vi "Set Value.vi"(7 "TOML string":string, 8 "error in (no error)":errorcluster, 9 "start position":i32, 10 "Value":T3, 11 "Context in":T2[](array[typedef])) -> (0 "error out":errorcluster, 1 "offset past match":i32, 2 "State":T1, 3 "Context out":T2[](array[typedef]))   [LabVIEW 2019, in "BlueTOMLSerializer.lvlib"]
uses:
  BlueTOMLSerializer.lvlib
  Value.ctl
  Key-Value Pair.ctl
  Table Context.ctl
  Table Array Context.ctl
  Array Context.ctl
  State.ctl
  <vilib>/regexp/Match Regular Expression.xnode
  Value Type.ctl
  Context.ctl
panel:
  in  "Define":bool=TRUE
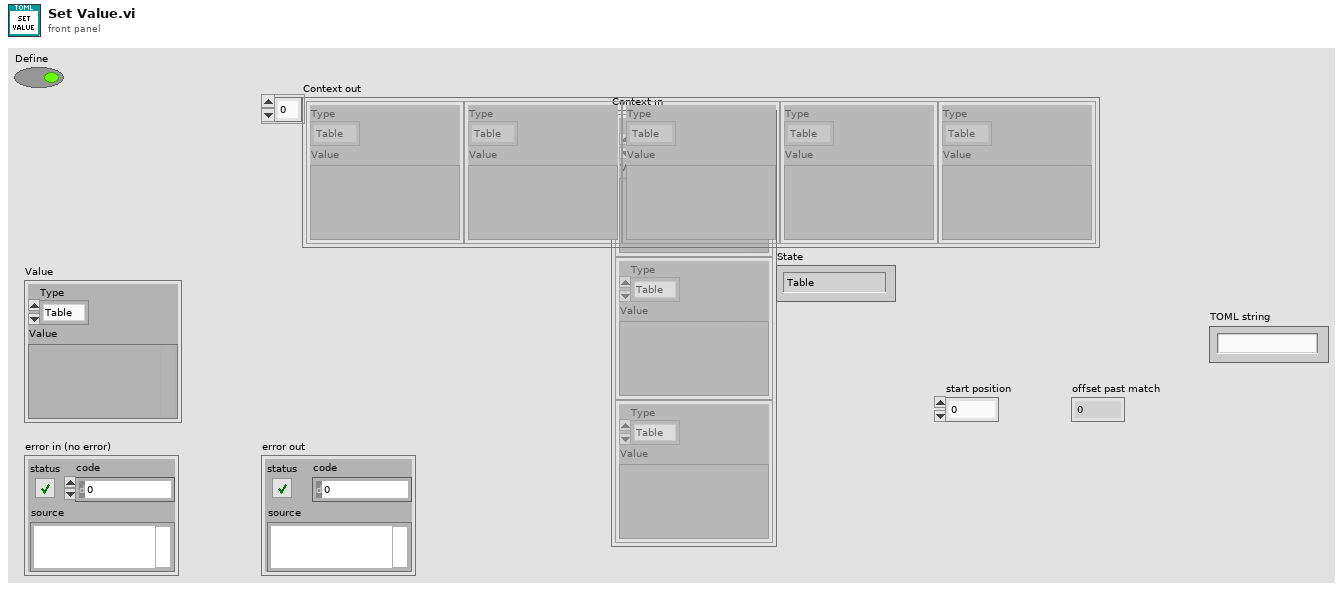
[diagram p1: front panel]
types:
  T1 = typedef "BlueTOMLSerializer.lvlib/State.ctl" = enum16{"Table", "Value", "Inline Table"}
  T2 = typedef "BlueTOMLSerializer.lvlib/Context.ctl" = cluster{"Type":enum16{"Table", "Array", "Inline Table", "Table Array"}, "Value":variant}
  T3 = typedef "BlueTOMLSerializer.lvlib/Value.ctl" = cluster{"Type":T4, "Value":variant}
  T4 = typedef "BlueTOMLSerializer.lvlib/Value Type.ctl" = enum16{"Table", "Array", "String", "Integer", "Float", "Boolean", "Offset Date-Time", "Local Date-Time", "Local Date", "Local Time"}
  T5 = typedef "BlueTOMLSerializer.lvlib/Table Context.ctl" = cluster{"Table":T6[], "Key":string, "Defined Keys":string[]}
  T6 = typedef "BlueTOMLSerializer.lvlib/Key-Value Pair.ctl" = cluster{"Key":string, "Value":T3}
  T7 = typedef "BlueTOMLSerializer.lvlib/Table Array Context.ctl" = cluster{"Table Array":cluster{"Table":T6[]}[], "Index":i32, "Key":string}
  T8 = typedef "BlueTOMLSerializer.lvlib/Array Context.ctl" = cluster{"Array":T3[], "Index":i32, "Empty":bool, "Type":T4}
  T9 = enum16{"Table", "Array", "Inline Table", "Table Array"}
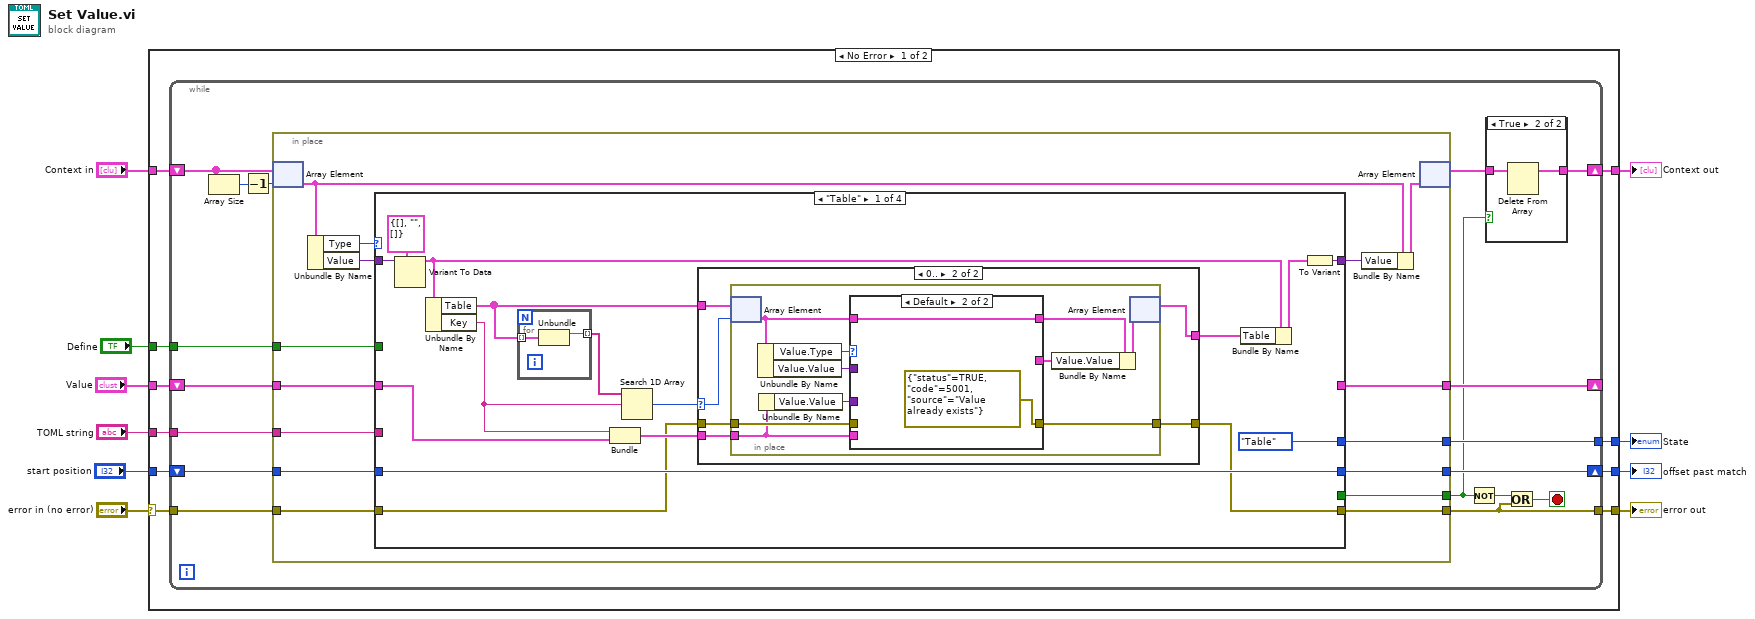
[diagram p0: block diagram]
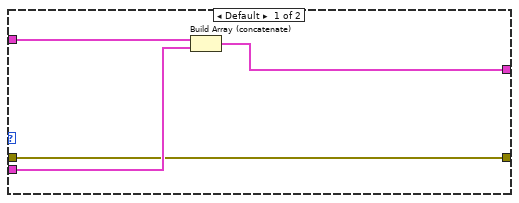
[diagram p3: hidden frame]
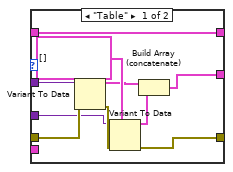
[diagram p4: hidden frame]
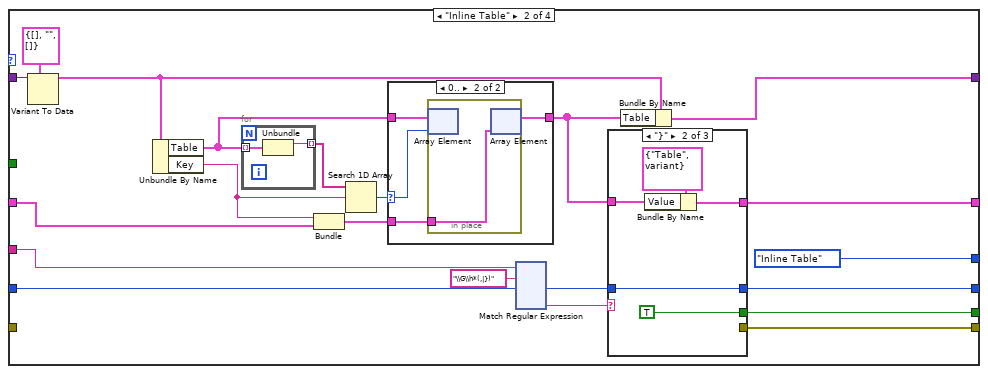
[diagram p5: hidden frame]
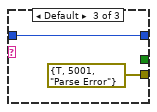
[diagram p7: hidden frame]
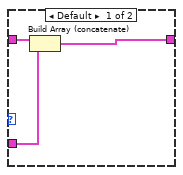
[diagram p8: hidden frame]
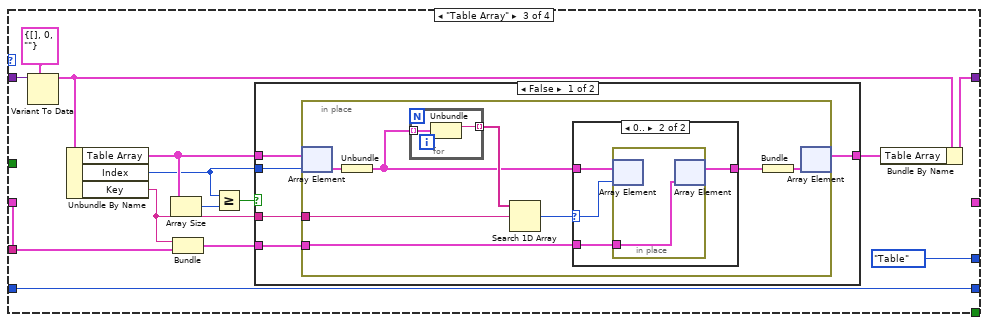
[diagram p9: hidden frame]
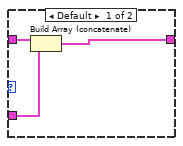
[diagram p10: hidden frame]
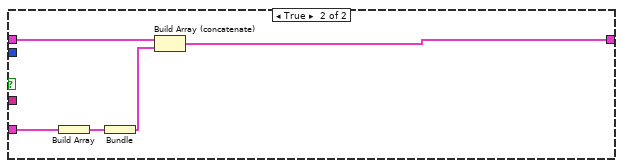
[diagram p11: hidden frame]
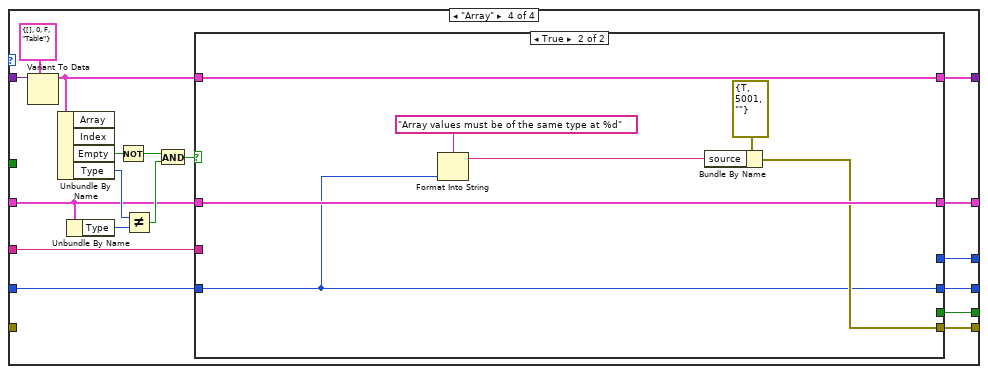
[diagram p12: hidden frame]
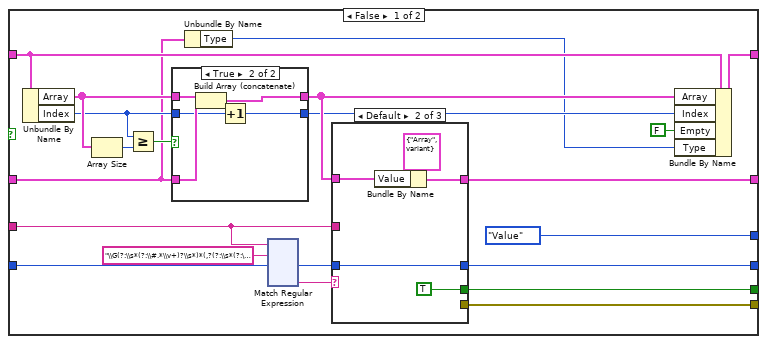
[diagram p13: hidden frame]
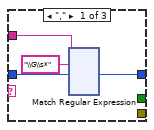
[diagram p14: hidden frame]
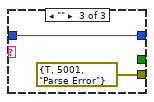
[diagram p15: hidden frame]
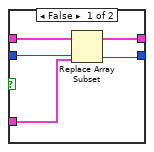
[diagram p16: hidden frame]
diagram:
  n1 = case shown="No Error" "error in (no error)" {
    selector: "error in (no error)" -> [w15 w603]
    tunnel: "Context in" -> [w20 w601]
    tunnel: [w19 w601] -> w9
    tunnel: "Value" -> [w18 _]
    tunnel: [w17 _] -> w7
    tunnel: [w16 w603] -> w6
    tunnel: "start position" -> [w14 w602]
    tunnel: "TOML string" -> [w13 _]
    tunnel: [w12 w602] -> w2
    tunnel: "Define" -> [w11 _]
    frame No Error {
      n2 = while {
        tunnel: [w33] -> w17
        tunnel: w13 -> [w28]
        shift-right: [w26] -> w12
        shift-left: w14 -> [w29]
        tunnel: w15 -> [w32]
        tunnel: [w30] -> w16
        shift-right: [w25] -> _
        shift-left: w18 -> [w34]
        shift-right: [w23] -> w19
        shift-left: w20 -> [w35]
        tunnel: w11 -> [w21]
        stop <- w31 stop-if-true
        n3 = Array Size(array=w35) -> (size(s)=w37:i32)
        n4 = Decrement(x=w37) -> (x-1=w36:i32)
        n5 = in-place {
          in-place-border: w34 -> [w50]
          in-place-border: [w49] -> w33
          in-place-border: [w48] -> w30
          in-place-border: w32 -> [w47]
          in-place-border: [w44] -> w22
          in-place-border: w29 -> [w46]
          in-place-border: w28 -> [w45]
          in-place-border: [w43] -> w25
          in-place-border: [w42] -> w26
          in-place-border: w21 -> [w41]
          n6 = in-place-array #1(w35, w36) -> (w53:T2)
          n7 = Unbundle By Name(w53) -> ("Type"=w55:T9, "Value"=w54:variant)
          n8 = case shown="\"Table\"" w55 {
            tunnel: w54 -> [w71 w126 w274 w320]
            tunnel: w50 -> [w65 w120 w270 w304]
            tunnel: [w60 w106 w263 w319] -> w52
            tunnel: [State."Table" ("State") State."Inline Table" ("State") State."Table" ("State") w317] -> w49
            tunnel: [w56 w107 _ w312] -> w48
            tunnel: w47 -> [w57 _ _ _]
            tunnel: w46 -> [w58 w116 w261 w315]
            tunnel: w45 -> [_ w115 _ w311]
            tunnel: [_ w111 _ w316] -> w44
            tunnel: [_ w109 _ w313] -> w43
            tunnel: [w58 w108 w261 w314] -> w42
            tunnel: w41 -> [_ _ _ _]
            frame "Table" {
              n9 = Variant To Data(type=T5 {"Table"=[], "Key"="", "Defined Keys"=[]} ("Table Context"), Variant=w71) -> (data=w64:T5)  [unwired: 1 in, 1 out]
              n10 = Unbundle By Name(w64) -> ("Table"=w67:T6[], "Key"=w66:string)
              n11 = for {
                tunnel: w67 -> [w105] mode=indexing
                tunnel: [w104] -> w69 mode=indexing
                n12 = Unbundle(w105) -> ("Key"=w104:string)  [unwired: 1 out]
              }
              n13 = Bundle("Key"=w66, "Value"=w65) -> (w61:cluster{"Key":string, "Value":T3})  [unwired: 1 in]
              n14 = Search 1D Array(1D array=w69, element=w66) -> (index of element=w68:i32)  [unwired: 1 in]
              n15 = case shown="0.." w68 {
                selector: w68 -> [_ w79]
                tunnel: w67 -> [w75 w81]
                tunnel: [w74 w80] -> w63
                tunnel: w61 -> [w73 w78]
                tunnel: w57 -> [w72 w77]
                tunnel: [w72 w76] -> w56
                frame Default {
                  n16 = Build Array (concatenate)(w75, w73) -> (w74:T6[])
                }
                frame 0.. {
                  n17 = in-place {
                    in-place-border: w78 -> [w84]
                    in-place-border: w77 -> [w86]
                    in-place-border: [w85] -> w76
                    n18 = in-place-array #2(w81, w79) -> (w90:T6)
                    n19 = Unbundle By Name(w90) -> ("Value.Type"=w89:T4, "Value.Value"=w88:variant)
                    n20 = Unbundle By Name(w84) -> ("Value.Value"=w83:variant)
                    n21 = case shown="Default" w89 {
                      tunnel: [w101 w103] -> w91
                      tunnel: w90 -> [w101 w103]
                      tunnel: w88 -> [w100 _]
                      tunnel: w84 -> [_ _]
                      tunnel: w86 -> [w99 _]
                      tunnel: [w93 errorcluster {"status"=TRUE, "code"=5001, "source"="Value already exists"} ("error constant")] -> w85
                      tunnel: w83 -> [w92 _]
                      tunnel: [w94 _] -> w82
                      frame "Table" {
                        w97 = T6[] []
                        n22 = Variant To Data(error in=w99, type=w97, Variant=w100) -> (data=w96:T6[], error out=w98:errorcluster)
                        n23 = Variant To Data(error in=w98, type=w97, Variant=w92) -> (data=w95:T6[], error out=w93:errorcluster)
                        n24 = Build Array (concatenate)(w96, w95) -> (w94:T6[])
                      }
                      frame Default {
                      }
                    }
                    n25 = Bundle By Name(cluster=w91, "Value.Value"=w82) -> (w87:T6)
                    n26 = in-place-array #2(w87) -> (w80:T6[])  [unwired: 1 out]
                  }
                }
              }
              n27 = Bundle By Name(cluster=w64, "Table"=w63) -> (w62:T5)
              n28 = To Variant(anything=w62) -> (Variant=w60:variant)
            }
            frame "Inline Table" {
              n29 = Variant To Data(type=T5 {"Table"=[], "Key"="", "Defined Keys"=[]} ("Table Context"), Variant=w126) -> (data=w119:T5)  [unwired: 1 in, 1 out]
              n30 = Unbundle By Name(w119) -> ("Table"=w122:T6[], "Key"=w121:string)
              n31 = for {
                tunnel: w122 -> [w260] mode=indexing
                tunnel: [w259] -> w124 mode=indexing
                n32 = Unbundle(w260) -> ("Key"=w259:string)  [unwired: 1 out]
              }
              n33 = Bundle("Key"=w121, "Value"=w120) -> (w118:cluster{"Key":string, "Value":T3})  [unwired: 1 in]
              n34 = Search 1D Array(1D array=w124, element=w121) -> (index of element=w123:i32)  [unwired: 1 in]
              n35 = case shown="0.." w123 {
                selector: w123 -> [_ w255]
                tunnel: w122 -> [w253 w257]
                tunnel: [w252 w256] -> w110
                tunnel: w118 -> [w251 w254]
                frame Default {
                  n36 = Build Array (concatenate)(w253, w251) -> (w252:T6[])
                }
                frame 0.. {
                  n37 = in-place {
                    in-place-border: w254 -> [w258]
                    n38 = in-place-array #3(w257, w255) -> ()  [unwired: 1 out]
                    n39 = in-place-array #3(w258) -> (w256:T6[])  [unwired: 1 out]
                  }
                }
              }
              n40 = xnode "Match Regular Expression"("input string"=w115, "regular expression"="\\G\\h*(,|})", "offset (0)"=w116) -> ("offset past match"=w112:i32, "submatch 1"=w113:string)  [unwired: 3 in, 4 out]
              n41 = case shown="\"}\"" w113 {
                tunnel: w112 -> [w243 w244 w250]
                tunnel: [_ TRUE _] -> w111
                tunnel: w110 -> [_ w246 _]
                tunnel: [_ w245 _] -> w109
                tunnel: [w243 w244 w250] -> w108
                tunnel: [_ _ errorcluster {"status"=TRUE, "code"=5001, "source"="Parse Error"} ("error constant")] -> w107
                frame "," {
                }
                frame "}" {
                  n42 = Bundle By Name(cluster=T3 {"Type"=enum."Table", "Value"=variant} ("Value"), "Value"=w246) -> (w245:T3)
                }
                frame Default {
                }
              }
              n43 = Bundle By Name(cluster=w119, "Table"=w110) -> (w106:T5)
            }
            frame "Table Array" {
              n44 = Variant To Data(type=T7 {"Table Array"=[], "Index"=0, "Key"=""} ("Table Array Context"), Variant=w274) -> (data=w267:T7)  [unwired: 1 in, 1 out]
              n45 = Unbundle By Name(w267) -> ("Table Array"=w268:cluster{"Table":T6[]}[], "Index"=w265:i32, "Key"=w264:string)
              n46 = Array Size(array=w268) -> (size(s)=w272:i32)
              n47 = Bundle("Key"=w264, "Value"=w270) -> (w269:cluster{"Key":string, "Value":T3})  [unwired: 1 in]
              n48 = Greater Or Equal?(x=w265, y=w272) -> (x >= y?=w271:bool)
              n49 = case shown="False" w271 {
                tunnel: w269 -> [w276 w302]
                tunnel: w268 -> [w279 w300]
                tunnel: [w275 w298] -> w266
                tunnel: w265 -> [w278 _]
                tunnel: w264 -> [w277 _]
                frame False {
                  n50 = in-place {
                    in-place-border: w277 -> [w282]
                    in-place-border: w276 -> [w281]
                    n51 = in-place-array #4(w279, w278) -> (w287:cluster{"Table":T6[]})
                    n52 = Unbundle(w287) -> ("Table"=w283:T6[])
                    n53 = for {
                      tunnel: w283 -> [w297] mode=indexing
                      tunnel: [w296] -> w285 mode=indexing
                      n54 = Unbundle(w297) -> ("Key"=w296:string)  [unwired: 1 out]
                    }
                    n55 = Search 1D Array(1D array=w285, element=w282) -> (index of element=w284:i32)  [unwired: 1 in]
                    n56 = case shown="0.." w284 {
                      selector: w284 -> [_ w292]
                      tunnel: w283 -> [w290 w294]
                      tunnel: [w289 w293] -> w280
                      tunnel: w281 -> [w288 w291]
                      frame Default {
                        n57 = Build Array (concatenate)(w290, w288) -> (w289:T6[])
                      }
                      frame 0.. {
                        n58 = in-place {
                          in-place-border: w291 -> [w295]
                          n59 = in-place-array #5(w294, w292) -> ()  [unwired: 1 out]
                          n60 = in-place-array #5(w295) -> (w293:T6[])  [unwired: 1 out]
                        }
                      }
                    }
                    n61 = Bundle("Table"=w280) -> (w286:cluster{"Table":T6[]})  [unwired: 1 in]
                    n62 = in-place-array #4(w286) -> (w275:cluster{"Table":T6[]}[])  [unwired: 1 out]
                  }
                }
                frame True {
                  n63 = Build Array(w302) -> (w301:cluster{"Key":string, "Value":T3}[])
                  n64 = Bundle(w301) -> (w299:cluster{cluster{"Key":string, "Value":T3}[]})  [unwired: 1 in]
                  n65 = Build Array (concatenate)(w300, w299) -> (w298:cluster{"Table":T6[]}[])
                }
              }
              n66 = Bundle By Name(cluster=w267, "Table Array"=w266) -> (w263:T7)
            }
            frame "Array" {
              n67 = Variant To Data(type=T8 {"Array"=[], "Index"=0, "Empty"=FALSE, "Type"=enum."Table"} ("Array Context"), Variant=w320) -> (data=w305:T8)  [unwired: 1 in, 1 out]
              n68 = Unbundle By Name(w305) -> ("Empty"=w310:bool, "Type"=w308:T4)  [unwired: 2 out]
              n69 = Unbundle By Name(w304) -> ("Type"=w309:T4)
              n70 = Not(x=w310) -> (.not. x?=w307:bool)
              n71 = Not Equal?(x=w308, y=w309) -> (x != y?=w306:bool)
              n72 = And(x=w307, y=w306) -> (x .and. y?=w303:bool)
              n73 = case shown="True" w303 {
                tunnel: [w339 w600] -> w319
                tunnel: [State."Value" ("State") _] -> w317
                tunnel: [w333 _] -> w316
                tunnel: w315 -> [w332 w594]
                tunnel: [w331 w594] -> w314
                tunnel: [w330 w599] -> w313
                tunnel: [w329 w595] -> w312
                tunnel: w311 -> [w327 _]
                tunnel: w305 -> [w325 w600]
                tunnel: w304 -> [w322 w599]
                frame False {
                  n74 = Unbundle By Name(w325) -> ("Array"=w324:T3[], "Index"=w323:i32)
                  n75 = Array Size(array=w324) -> (size(s)=w341:i32)
                  n76 = Greater Or Equal?(x=w323, y=w341) -> (x >= y?=w340:bool)
                  n77 = case shown="True" w340 {
                    tunnel: w324 -> [w588 w593]
                    tunnel: [w586 w592] -> w334
                    tunnel: w323 -> [w585 w590]
                    tunnel: w322 -> [w587 w591]
                    tunnel: [w585 w589] -> w328
                    frame False {
                      n78 = Replace Array Subset(array=w588, new element=w587, index=w585) -> (w586:T3[])
                    }
                    frame True {
                      n79 = Build Array (concatenate)(w593, w591) -> (w592:T3[])
                      n80 = Increment(x=w590) -> (x+1=w589:i32)
                    }
                  }
                  n81 = Unbundle By Name(w322) -> ("Type"=w321:T4)
                  n82 = xnode "Match Regular Expression"("input string"=w327, "regular expression"="\\G(?:\\s*(?:\\#.*\\v+)?\\s*)*(,?(?:\\s*(?:\\#.*\\v+)?\\s*)*\\]|,)", "offset (0)"=w332) -> ("offset past match"=w335:i32, "submatch 1"=w336:string)  [unwired: 3 in, 4 out]
                  n83 = case shown="Default" w336 {
                    tunnel: w335 -> [w459 w578 w584]
                    tunnel: [_ TRUE _] -> w333
                    tunnel: w334 -> [_ w580 _]
                    tunnel: [_ w579 _] -> w330
                    tunnel: [w458 w578 w584] -> w331
                    tunnel: [_ _ errorcluster {"status"=TRUE, "code"=5001, "source"="Parse Error"} ("error constant")] -> w329
                    tunnel: w327 -> [w460 _ _]
                    frame "," {
                      n84 = xnode "Match Regular Expression"("input string"=w460, "regular expression"="\\G\\s*", "offset (0)"=w459) -> ("offset past match"=w458:i32)  [unwired: 3 in, 5 out]
                    }
                    frame Default {
                      n85 = Bundle By Name(cluster=T3 {"Type"=enum."Array", "Value"=variant} ("Value"), "Value"=w580) -> (w579:T3)
                    }
                    frame "" {
                    }
                  }
                  n86 = Bundle By Name(cluster=w325, "Array"=w334, "Index"=w328, "Empty"=FALSE, "Type"=w321) -> (w339:T8)
                }
                frame True {
                  n87 = Format Into String(format string="Array values must be of the same type at %d", w594) -> (resulting string=w596:string)  [unwired: 2 in, 1 out]
                  n88 = Bundle By Name(cluster=errorcluster {"status"=TRUE, "code"=5001, "source"=""} ("error in (no error)"), "source"=w596) -> (w595:errorcluster)
                }
              }
            }
          }
          n89 = Bundle By Name(cluster=w53, "Value"=w52) -> (w51:T2)
          n90 = in-place-array #1(w51) -> (w24:T2[])  [unwired: 1 out]
        }
        n91 = Not(x=w22) -> (.not. x?=w27:bool)
        n92 = case shown="True" w22 {
          tunnel: w24 -> [w38 w40]
          tunnel: [w38 w39] -> w23
          frame False {
          }
          frame True {
            n93 = Delete From Array(array=w40) -> (array with subset deleted=w39:T2[])  [unwired: 2 in, 1 out]
          }
        }
        n94 = Or(x=w27, y=w30) -> (x .or. y?=w31:bool)
      }
    }
    frame Error {
    }
  }
  "error out" <- w6
  "Context out" <- w9
  "State" <- w7
  "offset past match" <- w2
